vi "EvaluateDataFlowBlock.vi"(8 "error in (no error)":errorcluster, 9 "data":T2, 10 "config in":T1, 11 "Qbus":refnum<class "Qbus.lvclass">) -> (0 "error out":errorcluster, 2 "config out":T1)   [LabVIEW 2017, in "IrDataEventCreator.lvlib"]
uses:
  <vilib>/addons/InsightCM/Devices/Shared/Ir/IrDataEventCreator/IrDataEventCreator.lvlib
  <vilib>/addons/InsightCM/Devices/Shared/Common/DataFlow/controls/Data.ctl
  <vilib>/addons/InsightCM/Utilities/DataAccessors/controls/wfmSGL_DVR.ctl
  <vilib>/addons/PointValueMap/controls/PointMap.ctl
  <vilib>/addons/InsightCM/Devices/Shared/Common/DataFlow/controls/Type.ctl
  <vilib>/addons/Qbus/Qbus.lvclass
  <vilib>/addons/InsightCM/Devices/Shared/Ir/IrDataEventCreator/controls/config.ctl
  <vilib>/addons/InsightCM/Devices/Shared/Ir/IrDataEventCreator/controls/IrDataEvent.ctl
  <vilib>/addons/InsightCM/Devices/Shared/Common/DataEvent/controls/EventReference.ctl
  <vilib>/addons/InsightCM/Devices/Shared/Common/DataEvent/controls/Event.ctl
  <vilib>/addons/InsightCM/MessageBus/Base/controls/DataEvent.ctl
  <vilib>/addons/InsightCM/MessageBus/Base/controls/KeyValuePair.ctl
  <vilib>/addons/InsightCM/Devices/Shared/Common/DataEvent/controls/DataSet.ctl
  <vilib>/addons/InsightCM/MessageBus/Base/controls/DataSetMetadata.ctl
  <vilib>/addons/InsightCM/MessageBus/Base/controls/TrendPoint.ctl
  <vilib>/addons/InsightCM/MessageBus/Base/controls/TrendAlarmUpdate.ctl
  <vilib>/addons/InsightCM/MessageBus/Base/controls/TrendAlarmTransition.ctl
  <vilib>/addons/PointValueMap/subVIs/Point_Read_string.vi
  <vilib>/addons/PointValueMap/PointValueMap.lvlib
  <vilib>/addons/InsightCM/Devices/Shared/Common/DataEvent/DataEvent.lvlib
  <vilib>/addons/InsightCM/Devices/Shared/Common/DataFlow/DataFlow.lvlib
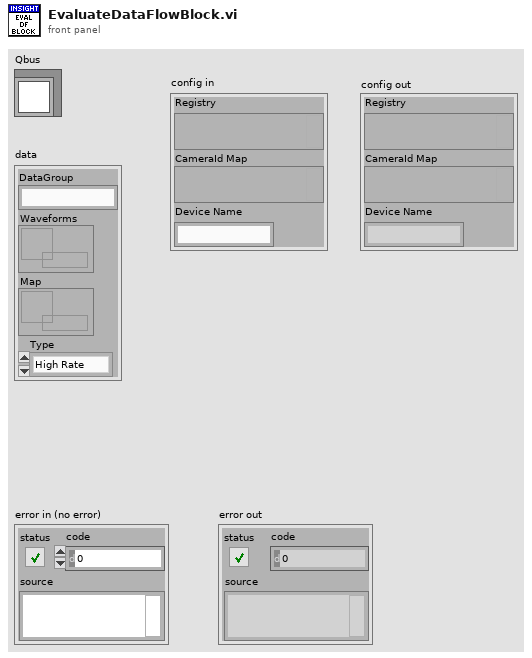
[diagram p1: front panel]
types:
  T1 = typedef "IrDataEventCreator.lvlib/config.ctl" = cluster{"Registry":variant, "CameraId Map":variant, "Device Name":string}
  T2 = typedef "DataFlow.lvlib/Data.ctl" = cluster{"DataGroup":string, "Waveforms":T3, "Map":T4, "Type":T5}
  T3 = typedef "wfmSGL_DVR.ctl" = refnum<data-value>
  T4 = typedef "PointValueMap.lvlib/PointMap.ctl" = refnum<data-value>
  T5 = typedef "DataFlow.lvlib/Type.ctl" = enum16{"High Rate", "Low Rate", "Burst Mode"}
  T6 = typedef "IrDataEventCreator.lvlib/IrDataEvent.ctl" = cluster{"event reference":T7, "OpState":string, "Reason":string, "Map":T4, "DataSetIds":variant, "IncludeImage":bool}
  T7 = typedef "DataEvent.lvlib/EventReference.ctl" = refnum<data-value>
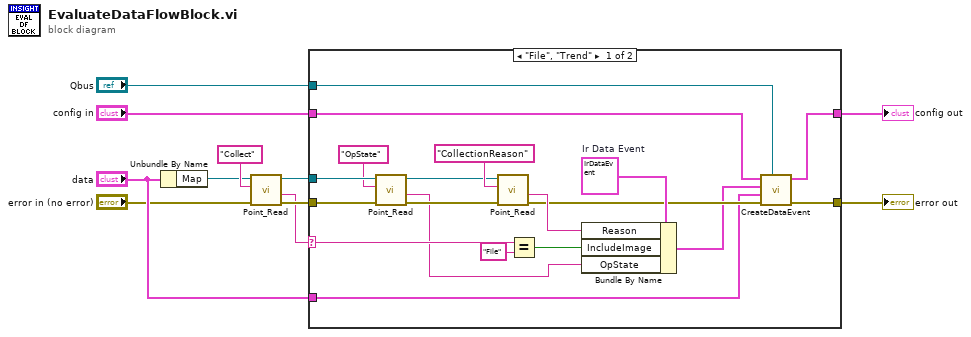
[diagram p0: block diagram]
diagram:
  n1 = Unbundle By Name("data") -> ("Map"=w2:T4)
  n2 = call-poly <vilib>:"Point_Read.vi"("Error In"="error in (no error)", "Tag"="Collect", "Map"=w2) -> ("Error Out"=w6:errorcluster, "Value"=w4:string, "Map Out"=w7:T4)  [unwired: 3 in, 3 out]
  n3 = case shown="\"File\", \"Trend\"" w4 {
    selector: w4 -> [w27 _]
    tunnel: w7 -> [w17 _]
    tunnel: w6 -> [w15 w32]
    tunnel: [w25 w32] -> w11
    tunnel: "config in" -> [w21 w31]
    tunnel: "Qbus" -> [w19 _]
    tunnel: "data" -> [w22 _]
    tunnel: [w20 w31] -> w3
    frame "File", "Trend" {
      w28 = T6 {"event reference"=refnum, "OpState"="", "Reason"="", "Map"=refnum, "DataSetIds"=variant, "IncludeImage"=FALSE}  # Ir Data Event
      n4 = call-poly <vilib>:"Point_Read.vi"("Error In"=w15, "Tag"="OpState", "Map"=w17) -> ("Error Out"=w14:errorcluster, "Value"=w12:string, "Map Out"=w16:T4)  [unwired: 3 in, 3 out]
      n5 = call-poly <vilib>:"Point_Read.vi"("Error In"=w14, "Tag"="CollectionReason", "Map"=w16) -> ("Error Out"=w24:errorcluster, "Value"=w29:string)  [unwired: 3 in, 4 out]
      n6 = Equal?(x=w27, y="File") -> (x = y?=w18:bool)
      n7 = Bundle By Name(cluster=w28, "Reason"=w29, "IncludeImage"=w18, "OpState"=w12) -> (w23:T6)
      n8 = call <vilib>:"CreateDataEvent.vi"("Qbus"=w19, "error in (no error)"=w24, "data"=w22, "Ir Data Event"=w23, "config in"=w21) -> ("error out"=w25:errorcluster, "config out"=w20:T1)  [unwired: 5 in]
    }
    frame Default {
    }
  }
  "error out" <- w11
  "config out" <- w3
